vi "SGL Complex to 64-bit Number.vi"(7 "Input CSG":T1) -> (8 "64-bit Complex":u64)   [LabVIEW 2011]
types:
  T1 = cluster{"xk_im":fxp<+,32,32>, "xk_re":fxp<+,32,32>}
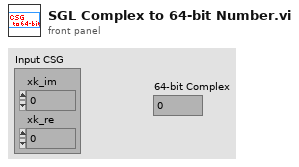
[diagram p1: front panel]
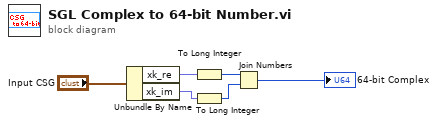
[diagram p0: block diagram]
diagram:
  n1 = Unbundle By Name("Input CSG") -> ("xk_re"=w6:fxp<+,32,32>, "xk_im"=w5:fxp<+,32,32>)
  n2 = To Long Integer(number=w6) -> (32bit integer=w4:i32)
  n3 = To Long Integer(number=w5) -> (32bit integer=w2:i32)
  n4 = Join Numbers(hi=w4, lo=w2) -> ((hi.lo)=→"64-bit Complex":u64)
